vi "Split DMA by Direction.vi"(11 "DMA configuration array":T1[](array[typedef])) -> (2 "HostToTarget":T1[](array[typedef]), 3 "TargetToHost":T1[](array[typedef]))   [LabVIEW 2013, in "FPGA Addon System Explorer.lvlib"]
uses:
  FPGA Addon System Explorer.lvlib
  <vilib>/rvi/FIFO/Fifo_Types/Fifo_DMA_Config.ctl
  <vilib>/rvi/DataTransferAndStorage/Container/Common/niFpgaDataTypeControl.ctl
  <vilib>/rvi/ClientSDK/Core/ModuleGeneration/CommunicationInterfaceUtility/niFpgaDmaChannelImplementation.ctl
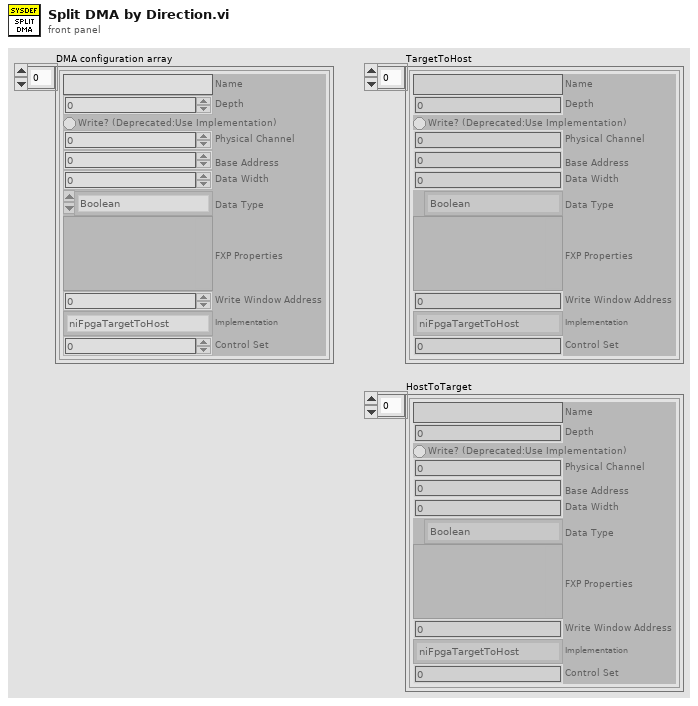
[diagram p1: front panel]
types:
  T1 = typedef "Fifo_DMA_Config.ctl" = cluster{"Name":string, "Depth":u32, "Write? (Deprecated:Use Implementation)":bool, "Physical Channel":u32, "Base Address":u32, "Data Width":u32, "Data Type":T2, "FXP Properties":variant, "Write Window Address":u32, "Implementation":T3, "Control Set":u32}
  T2 = typedef "niFpgaDataTypeControl.ctl" = enum32{"Boolean", "I8", "I16", "I32", "I64", "U8", "U16", "U32", "U64", "FXP", "CustomControl", "SGL"}
  T3 = typedef "niFpgaDmaChannelImplementation.ctl" = enum16{"niFpgaTargetToHost", "niFpgaHostToTarget", "niFpgaPeerToPeerWriter", "niFpgaPeerToPeerReader", "niCoreTargetToHost", "niCoreHostToTarget"}
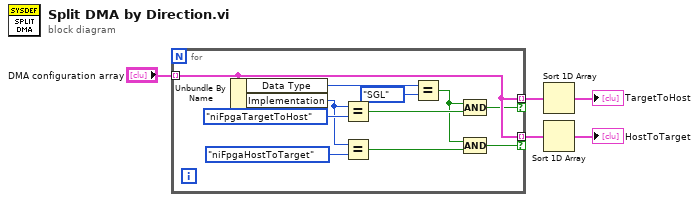
[diagram p0: block diagram]
diagram:
  n1 = for {
    tunnel: "DMA configuration array" -> [w12] mode=indexing
    tunnel: [w12] -> w1 mode=indexing if=w9
    tunnel: [w12] -> w3 mode=indexing if=w6
    n2 = Unbundle By Name(w12) -> ("Data Type"=w11:T2, "Implementation"=w15:T3)
    n3 = Equal?(x=w15, y=niFpgaDmaChannelImplementation."niFpgaTargetToHost") -> (x = y?=w13:bool)
    n4 = Equal?(x=w15, y=niFpgaDmaChannelImplementation."niFpgaHostToTarget") -> (x = y?=w7:bool)
    n5 = Equal?(x=w11, y=niFpgaDataTypeControl."SGL") -> (x = y?=w8:bool)
    n6 = Compound Arithmetic op=AND(w8, w13) -> (w9:bool)
    n7 = Compound Arithmetic op=AND(w8, w7) -> (w6:bool)
  }
  n8 = Sort 1D Array(array=w1) -> (sorted array=→"TargetToHost":T1[])
  n9 = Sort 1D Array(array=w3) -> (sorted array=→"HostToTarget":T1[])
